vi "Divide by Gain.vi"(8 "error in (no error)":errorcluster, 10 "Gain":dbl[](array[numeric]), 11 "WFM in":waveform(dbl)[](array[waveform])) -> (0 "error out":errorcluster, 3 "WFM out":waveform(dbl)[](array[waveform]))   [LabVIEW 2016, in "Instrument.Lockin.lvclass"]
uses:
  Instrument.Lockin.lvclass
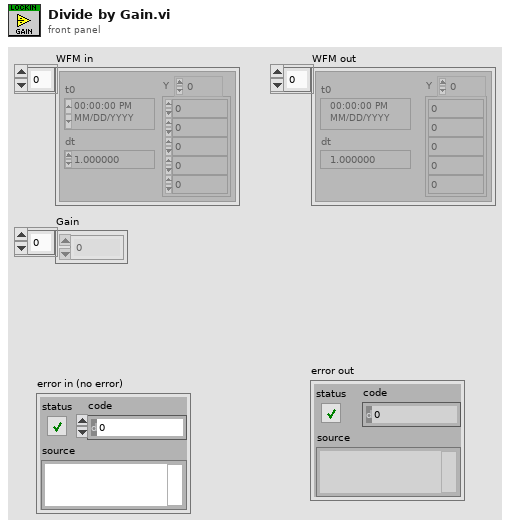
[diagram p1: front panel]
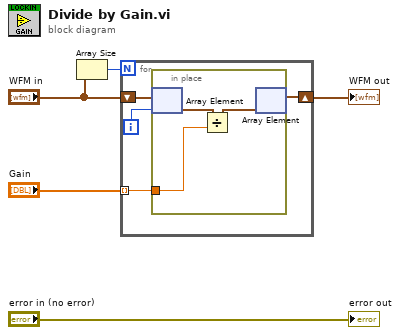
[diagram p0: block diagram]
diagram:
  n1 = Array Size(array="WFM in") -> (size(s)=w5:i32)
  n2 = for {
    N: w5 -> [_]
    shift-right: [w7] -> w4
    shift-left: "WFM in" -> [w8]
    tunnel: "Gain" -> [w6] mode=indexing
    i -> [w9]
    n3 = in-place {
      in-place-border: w6 -> [w11]
      n4 = in-place-array #1(w8, w9) -> (w12:waveform(dbl))
      n5 = Divide(x=w12, y=w11) -> (x/y=w10:waveform(dbl))
      n6 = in-place-array #1(w10) -> (w7:waveform(dbl)[])  [unwired: 1 out]
    }
  }
  "WFM out" <- w4
  "error out" <- "error in (no error)"
